vi "Init.vi"(8 "error in (no error)":errorcluster, 9 "ConfigurationJSON":string, 10 "Address":string, 11 "RMXPowerSupply in":refnum<class "RMXPowerSupply.lvclass">) -> (0 "error out":errorcluster, 1 "RunningInformation":string, 2 "Status":i32, 3 "RMXPowerSupply out":refnum<class "RMXPowerSupply.lvclass">, 4 "ErrorCode":i32)   [LabVIEW 2023, in "RMXPowerSupply.lvclass"]
uses:
  RMXPowerSupply.lvclass
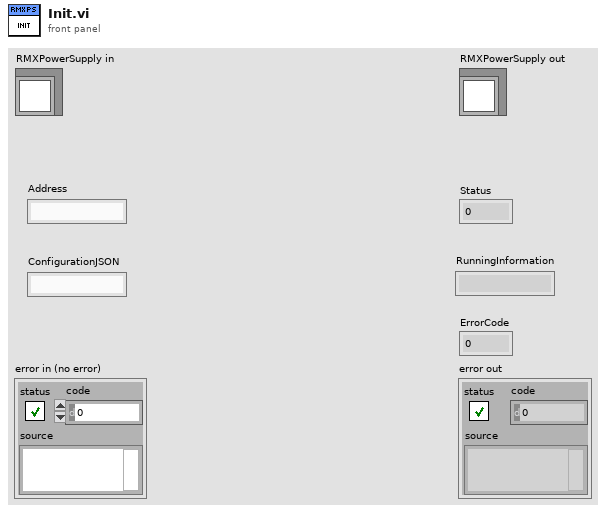
[diagram p1: front panel]
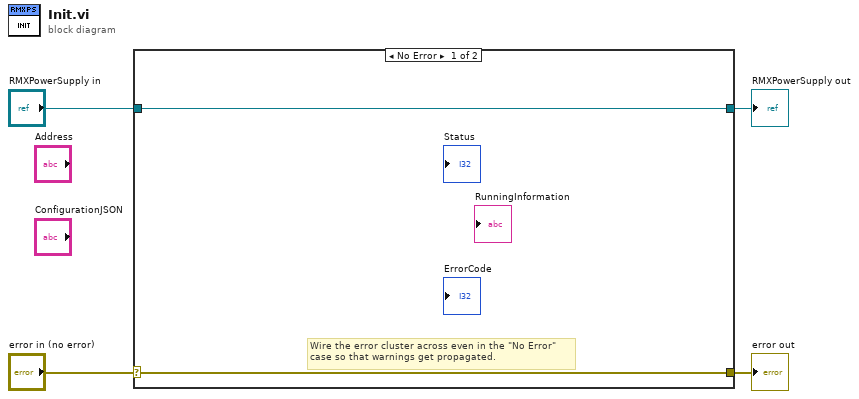
[diagram p0: block diagram]
diagram:
  n1 = case shown="No Error" "error in (no error)" {
    selector: "error in (no error)" -> [w5 w8]
    tunnel: [w5 w8] -> w3
    tunnel: [w6 w7] -> w1
    tunnel: "RMXPowerSupply in" -> [w6 w7]
    frame No Error {
      # "Wire the error cluster across even in the \"No Error\"\ncase so that warnings get propagated."
    }
    frame Error {
    }
  }
  "error out" <- w3
  "RMXPowerSupply out" <- w1
